vi "EditorThumbnail mouseUp.vi"(8 "error in (no error)":errorcluster, 11 "EditorThumbnail in":refnum<class "EditorThumbnail.lvclass">) -> (0 "error out":errorcluster, 3 "EditorThumbnail out":refnum<class "EditorThumbnail.lvclass">)   [LabVIEW 2018, in "EditorThumbnail.lvclass"]
uses:
  EditorThumbnail.lvclass
  EditorThumbnail.lvclass/EditorThumbnail.ctl
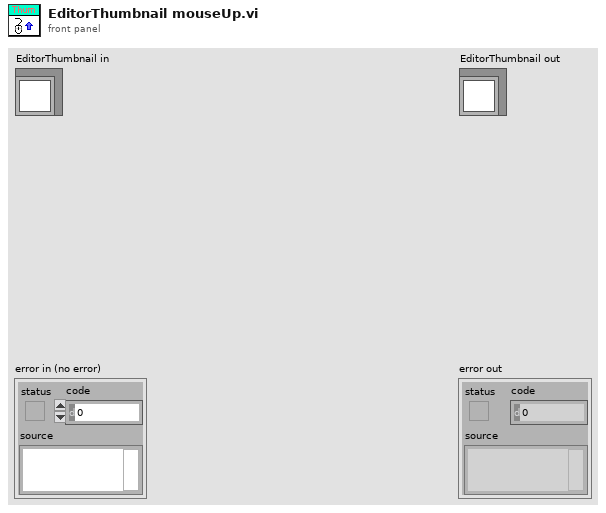
[diagram p1: front panel]
types:
  T1 = cluster{"index":u32, "data":cluster{"xdata":dbl[], "ydata":sgl[]}[], "peak":dbl[], "picture":picture}[]
  T2 = cluster{"index":u32, "data":cluster{"xdata":dbl[], "ydata":sgl[]}[], "peak":dbl[], "picture":picture}
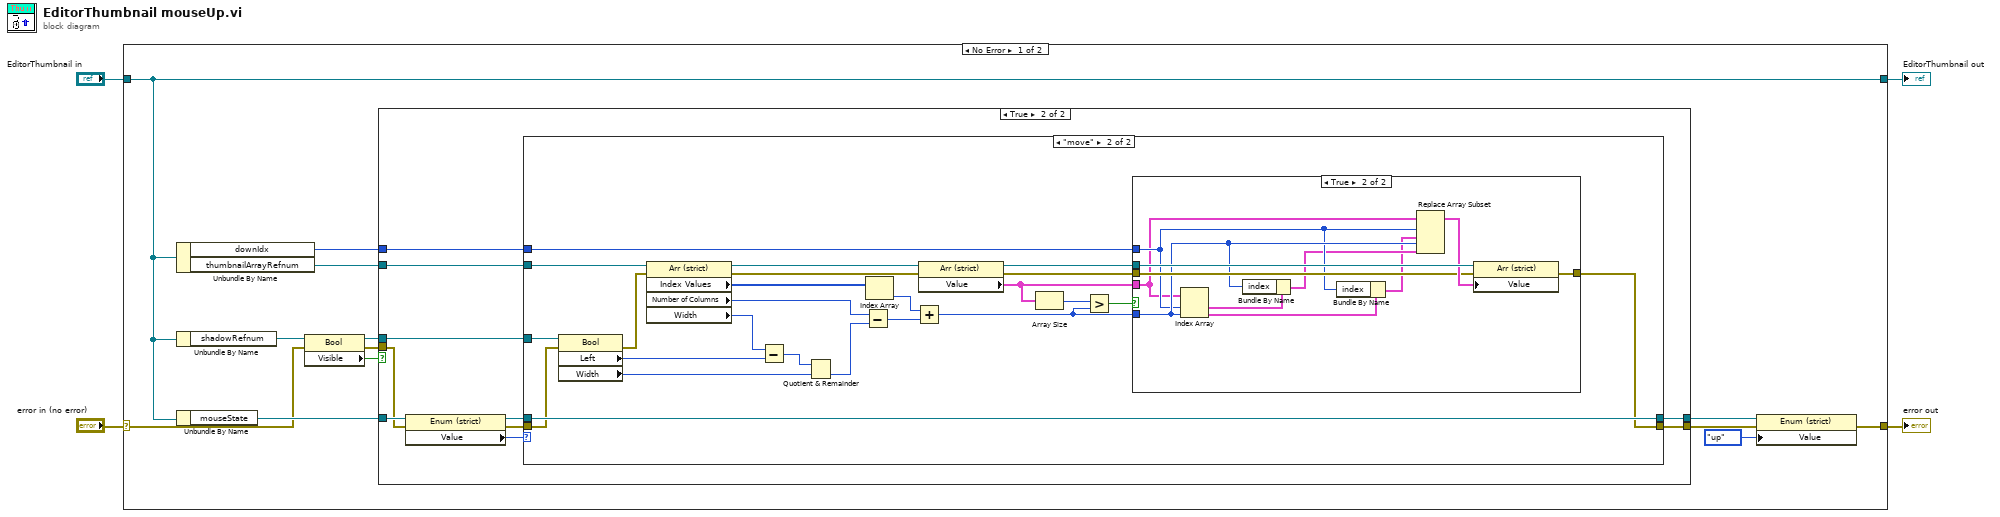
[diagram p0: block diagram]
diagram:
  n1 = case shown="No Error" "error in (no error)" {
    selector: "error in (no error)" -> [w7 w69]
    tunnel: [w10 w69] -> w3
    tunnel: [w12 w68] -> w1
    tunnel: "EditorThumbnail in" -> [w12 w68]
    frame No Error {
      n2 = Unbundle By Name(w12) -> ("downIdx"=w14:i32, "thumbnailArrayRefnum"=w16:refnum<vi>)
      n3 = Unbundle By Name(w12) -> ("shadowRefnum"=w9:refnum<vi>)
      n4 = Unbundle By Name(w12) -> ("mouseState"=w13:refnum<vi>)
      n5 = property class="Bool"(reference=w9, error in=w7) -> (reference out=w8:refnum<vi>, error out=w6:errorcluster, "Visible"=w5:bool)
      n6 = case shown="True" w5 {
        tunnel: w16 -> [_ w29]
        tunnel: [w18 w28] -> w15
        tunnel: w14 -> [_ w27]
        tunnel: w13 -> [w19 w26]
        tunnel: [w19 w24] -> w11
        tunnel: w8 -> [_ w21]
        tunnel: w6 -> [w18 w20]
        frame False {
        }
        frame True {
          n7 = property class="Enum (strict)"(reference=w26, error in=w20) -> (reference out=w23:refnum<vi>, error out=w22:errorcluster, "Value"=w25:enum16{"idle", "down", "move", "up"})
          n8 = case shown="\"move\"" w25 {
            tunnel: w21 -> [_ w55]
            tunnel: w29 -> [_ w52]
            tunnel: [w30 w38] -> w28
            tunnel: w27 -> [_ w36]
            tunnel: [w31 w43] -> w24
            tunnel: w23 -> [w31 w43]
            tunnel: w22 -> [w30 w42]
            frame "idle", Default {
            }
            frame "move" {
              n9 = property class="Bool"(reference=w55, error in=w42) -> (error out=w37:errorcluster, "Left"=w54:i32, "Width"=w49:u32)  [unwired: 1 out]
              n10 = property class="Arr (strict)"(reference=w52, error in=w37) -> (reference out=w44:refnum<vi>, error out=w40:errorcluster, "Index Values"=w47:u32[], "Number of Columns"=w50:u32, "Width"=w48:u32)
              n11 = Subtract(x=w48, y=w54) -> (x-y=w53:u32)
              n12 = Quotient & Remainder(x=w53, y=w49) -> (floor(x/y)=w51:u32)  [unwired: 1 out]
              n13 = Subtract(x=w50, y=w51) -> (x-y=w45:u32)
              n14 = Index Array(array=w47) -> (element=w46:u32)  [unwired: 1 in]
              n15 = Add(x=w46, y=w45) -> (x+y=w33:u32)
              n16 = property class="Arr (strict)"(reference=w44, error in=w40) -> (reference out=w41:refnum<vi>, error out=w39:errorcluster, "Value"=w35:T1)
              n17 = Array Size(array=w35) -> (size(s)=w34:i32)
              n18 = Greater?(x=w34, y=w33) -> (0:w32:bool)
              n19 = case shown="True" w32 {
                tunnel: w41 -> [_ w67]
                tunnel: w39 -> [w56 w65]
                tunnel: [w56 w64] -> w38
                tunnel: w33 -> [_ w61]
                tunnel: w36 -> [_ w60]
                tunnel: w35 -> [_ w57]
                frame False {
                }
                frame True {
                  n20 = Index Array(array=w57, index #1=w60, index #2=w61) -> (element #1=w63:T2, element #2=w62:T2)
                  n21 = Bundle By Name(cluster=w63, "index"=w61) -> (w59:T2)
                  n22 = Bundle By Name(cluster=w62, "index"=w60) -> (w58:T2)
                  n23 = Replace Array Subset(array=w57, new element #1=w58, index #1=w60, new element #2=w59, index #2=w61) -> (w66:T1)
                  n24 = property class="Arr (strict)"(reference=w67, error in=w65, "Value"=w66) -> (error out=w64:errorcluster)  [unwired: 1 out]
                }
              }
            }
          }
        }
      }
      n25 = property class="Enum (strict)"(reference=w11, error in=w15, "Value"=enum16{"idle", "down", "move", "up"}."up") -> (error out=w10:errorcluster)  [unwired: 1 out]
    }
    frame Error {
    }
  }
  "error out" <- w3
  "EditorThumbnail out" <- w1
